vi "Adv_WriteLightFieldProperty.vi"(8 "error in (no error)":errorcluster, 9 "value":refnum<k24>, 10 "setting":string, 11 "LightField Automation in":refnum<class "LightField Automation.lvclass">) -> (0 "error out":errorcluster, 3 "LightField Automation out":refnum<class "LightField Automation.lvclass">)   [LabVIEW 2015, in "LightField Automation.lvclass"]
uses:
  LightField Automation.lvclass
  LightField Automation.lvclass/LightField Automation.ctl
  C:/Program Files/Princeton Instruments/LightField/AddInViews/PrincetonInstruments.LightFieldViewV3.dll
  Program Files/Princeton Instruments/LightField/AddInViews/PrincetonInstruments.LightFieldViewV3.dll
  <vilib>/Utility/error.llb/DialogType.ctl
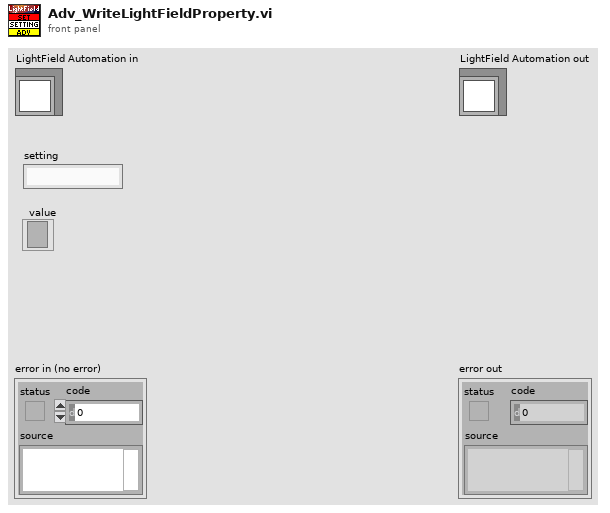
[diagram p1: front panel]
types:
  T1 = typedef "DialogType.ctl" = u16
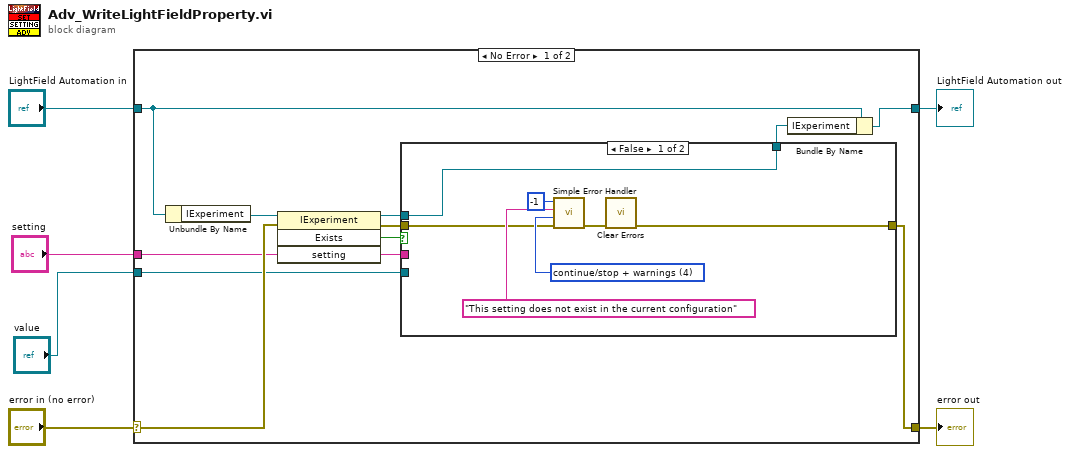
[diagram p0: block diagram]
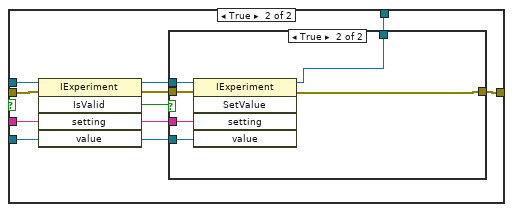
[diagram p2: hidden frame]
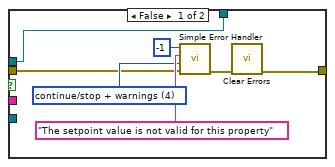
[diagram p3: hidden frame]
diagram:
  n1 = case shown="No Error" "error in (no error)" {
    selector: "error in (no error)" -> [w15 w48]
    tunnel: [w17 w48] -> w5
    tunnel: [w8 w47] -> w3
    tunnel: "LightField Automation in" -> [w9 w47]
    tunnel: "setting" -> [w11 _]
    tunnel: "value" -> [w10 _]
    frame No Error {
      n2 = Unbundle By Name(w9) -> ("IExperiment"=w16:refnum<k24>)
      n3 = invoke class="IExperiment" method="Exists"(reference=w16, error in=w15, "setting"=w11) -> (reference out=w13:refnum<k24>, error out=w12:errorcluster, "Exists"=w14:bool)  [unwired: 1 in, 1 out]
      n4 = case shown="False" w14 {
        tunnel: [w21 w33] -> w17
        tunnel: w13 -> [w18 w32]
        tunnel: w12 -> [w19 w31]
        tunnel: w11 -> [_ w27]
        tunnel: w10 -> [_ w26]
        tunnel: [w18 w25] -> w7
        frame False {
          w20 = T1 4 items=["no dialog", "OK message", "continue or stop message", "OK message + warnings", "continue/stop + warnings"] ("type of dialog (OK msg:1)")
          n5 = call <vilib>:"Simple Error Handler.vi"("error code (no error:0)"=-1, "error source (\" \")"="This setting does not exist in the current configuration" ("source"), "type of dialog (OK msg:1)"=w20, "error in (no error)"=w19) -> ("error out"=w22:errorcluster)  [unwired: 1 in, 4 out]
          n6 = call <vilib>:"Clear Errors.vi"("error in (no error)"=w22) -> ("error out"=w21:errorcluster)  [unwired: 5 in, 1 out]
        }
        frame True {
          n7 = invoke class="IExperiment" method="IsValid"(reference=w32, error in=w31, "setting"=w27, "value"=w26) -> (reference out=w29:refnum<k24>, error out=w28:errorcluster, "IsValid"=w30:bool)  [unwired: 1 in, 2 out]
          n8 = case shown="True" w30 {
            tunnel: [w38 w42] -> w33
            tunnel: w29 -> [w34 w46]
            tunnel: w28 -> [w35 w45]
            tunnel: w27 -> [_ w44]
            tunnel: w26 -> [_ w43]
            tunnel: [w34 w41] -> w25
            frame False {
              w36 = T1 4 items=["no dialog", "OK message", "continue or stop message", "OK message + warnings", "continue/stop + warnings"] ("type of dialog (OK msg:1)")
              n9 = call <vilib>:"Simple Error Handler.vi"("error code (no error:0)"=-1, "error source (\" \")"="The setpoint value is not valid for this property" ("source"), "type of dialog (OK msg:1)"=w36, "error in (no error)"=w35) -> ("error out"=w39:errorcluster)  [unwired: 1 in, 4 out]
              n10 = call <vilib>:"Clear Errors.vi"("error in (no error)"=w39) -> ("error out"=w38:errorcluster)  [unwired: 5 in, 1 out]
            }
            frame True {
              n11 = invoke class="IExperiment" method="SetValue"(reference=w46, error in=w45, "setting"=w44, "value"=w43) -> (reference out=w41:refnum<k24>, error out=w42:errorcluster)  [unwired: 1 in, 3 out]
            }
          }
        }
      }
      n12 = Bundle By Name(cluster=w9, "IExperiment"=w7) -> (w8:refnum<class "LightField Automation.lvclass">)
    }
    frame Error {
    }
  }
  "error out" <- w5
  "LightField Automation out" <- w3
